vi "Fetch (Internal Buffer).vi"(8 "error in (no error)":errorcluster, 9 "Timeout (10000 ms)":u32=10000, 11 "VISA resource name":refnum<visa-resource-name>) -> (0 "error out":errorcluster, 2 "Measurements":dbl[](array[numeric]), 3 "VISA resource name out":refnum<visa-resource-name>)   [LabVIEW 2015, in "Agilent 34401.lvlib"]
doc: "This low level VI transfers readings from the instrument's internal memory buffer to the output buffer and returns an array of values from the previously initiated measurement. The number of measurements the DMM takes is determined by the values you specify for the Trigger Count and Sample Count of the <B>Configure Multipoint VI</B>.\n\nThis VI is intended to be used in conjunction with the <B>Initiate (Internal Buffer) VI</B>.\n\n<B>Note:</B>\n\n(1) This VI has been obsoleted from the driver and is included for compatibility with existing applications. New applications should use the <B>Fetch Measurement VI</B>.\n\n(2) This VI does not check the instrument status. Typically, you call this VI only in a sequence of calls to other low-level instrument driver VIs. The sequence performs one operation. You use the low-level VIs to optimize one or more aspects of interaction with the instrument. If you want to check the instrument status, call the <B>Error Query VI</B> at the conclusion of the sequence."
uses:
  <instrlib>/Agilent 34401/Agilent 34401.lvlib
panel:
  # "Note:\nThis VI has been obsoleted from the driver and is included for compatibility with existing applications.  New applications should use the Fetch Measurement VI."
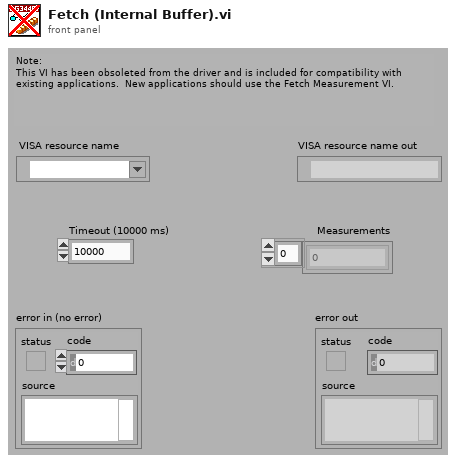
[diagram p1: front panel]
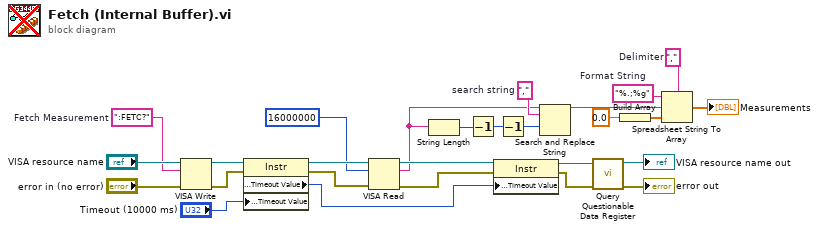
[diagram p0: block diagram]
diagram:
  w11 = ","  # search string
  w14 = ","  # Delimiter
  w15 = "%.;%g"  # Format String
  w25 = ":FETC?"  # Fetch Measurement
  n1 = VISA Write(VISA resource name="VISA resource name", write buffer=w25, error in (no error)="error in (no error)") -> (VISA resource name out=w24:refnum<visa-resource-name>, error out=w23:errorcluster)  [unwired: 1 out]
  n2 = property on="Property Node" class="Instr"(reference=w24, error in=w23, "General Settings:Timeout Value"="Timeout (10000 ms)") -> (reference out=w22:refnum<visa-resource-name>, error out=w21:errorcluster, "General Settings:Timeout Value"=w17:u32)
  n3 = VISA Read(VISA resource name=w22, byte count=u32 16000000, error in (no error)=w21) -> (VISA resource name out=w19:refnum<visa-resource-name>, read buffer=w7:string, error out=w18:errorcluster)  [unwired: 1 out]
  n4 = String Length(string=w7) -> (length=w5:i32)
  n5 = Decrement(x=w5) -> (x-1=w6:i32)
  n6 = property on="Property Node" class="Instr"(reference=w19, error in=w18, "General Settings:Timeout Value"=w17) -> (reference out=w1:refnum<visa-resource-name>, error out=w2:errorcluster)
  n7 = Decrement(x=w6) -> (x-1=w9:i32)
  n8 = Search and Replace String(input string=w7, search string=w11, offset=w9) -> (result string=w10:string)  [unwired: 5 in, 3 out]
  n9 = call <instrlib>:"Query Questionable Data Register.vi"("error in (no error)"=w2, "VISA resource name"=w1) -> ("error out"=→"error out":errorcluster, "VISA resource name out"=→"VISA resource name out":refnum<visa-resource-name>)  [unwired: 7 in, 1 out]
  n10 = Build Array(0.0) -> (w12:dbl[])
  n11 = Spreadsheet String To Array(delimiter (Tab)=w14, format string=w15, spreadsheet string=w10, array type (2D Dbl)=w12) -> (array=→"Measurements":dbl[])
